vi "Add To DAQmx Task.vi"(6 "Ignore Cal? (F)":bool, 7 "RTD in":refnum<class "RTD.lvclass">, 8 "error in (no error)":errorcluster, 9 "Scale Name":string, 10 "Chassis Name":string, 11 "task in":refnum<k21>) -> (0 "error out":errorcluster, 2 "Phys Chan Added":string, 3 "task out":refnum<k21>)   [LabVIEW 2018, in "Measurement Channels.lvlib" / "RTD.lvclass"]
uses:
  RTD.lvclass
  C:/Users/Jeff Tipps/Documents/DAQMan/source/Classes/Measurements/Class Channel/Channel.lvclass
  RTD.lvclass/RTD.ctl
  Class Channel/Read ChanName.vi
  Class Channel/Read Alias.vi
  <vilib>/DAQmx/create/channels.llb/DAQmx Create Channel (AI-Temperature-RTD).vi
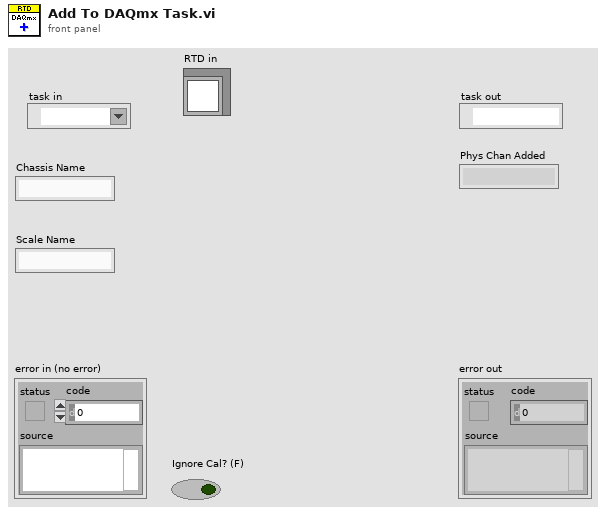
[diagram p1: front panel]
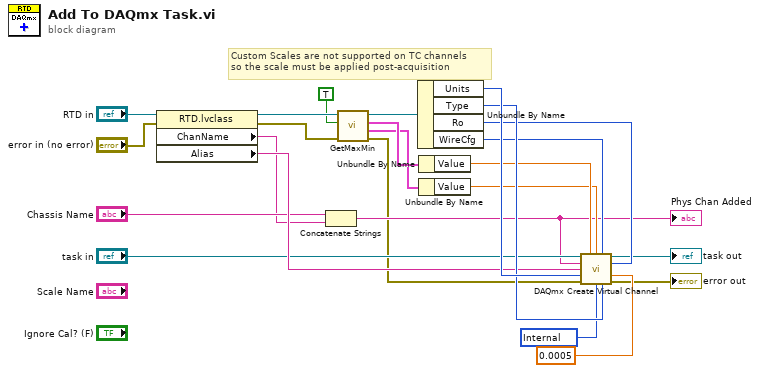
[diagram p0: block diagram]
diagram:
  w20 = 10200 items=["Internal"=10200, "External"=10167, "None"=10230] ("current excitation source")
  # "Custom Scales are not supported on TC channels\nso the scale must be applied post-acquisition"
  n1 = property class="RTD.lvclass"(reference="RTD in", error in="error in (no error)") -> (reference out=w16:refnum<class "RTD.lvclass">, error out=w14:errorcluster, "ChanName"=w5:string, "Alias"=w15:string)
  n2 = Concatenate Strings("Chassis Name", w5) -> (w4:string)
  "Phys Chan Added" <- w4
  n3 = call-dynamic "GetMaxMin.vi"("error in (no error)"=w14, "Ignore Cal? (F)"=TRUE, "RTD in"=w16) -> ("error out"=w2:errorcluster, "Min"=w8:cluster{"Value":dbl, "Text":string}, "Max"=w10:cluster{"Value":dbl, "Text":string}, "RTD out"=w18:refnum<class "RTD.lvclass">)  [unwired: 5 in]
  n4 = Unbundle By Name(w18) -> ("Units"=w24:u16, "Type"=w23:u16, "Ro"=w22:u16, "WireCfg"=w19:u16)
  n5 = Unbundle By Name(w10) -> ("Value"=w9:dbl)
  n6 = Unbundle By Name(w8) -> ("Value"=w7:dbl)
  n7 = call-poly <vilib>:"DAQmx Create Virtual Channel.vi"("task in"="task in", "maximum value"=w9, "minimum value"=w7, "resistance configuration"=w19, "physical channels"=w4, "r0"=w22, "name to assign"=w15, "units"=w24, "current excitation value"=0.0005, "error in"=w2, "current excitation source"=w20, "rtd type"=w23) -> ("task out"=→"task out":refnum<k21>, "error out"=→"error out":errorcluster)  [unwired: 2 in]
